vi "Global Parameter.vi"(3 "error in (no error)":errorcluster caption="错误输入（无错误）", 4 "Write":T1, 5 "枚举":enum16{"Inital", "Read", "Write", "Quit"}(ring)) -> (0 "错误输出":errorcluster, 1 "Read":T1)   [LabVIEW 2023]
uses:
  Ctl/Global Parameter.ctl
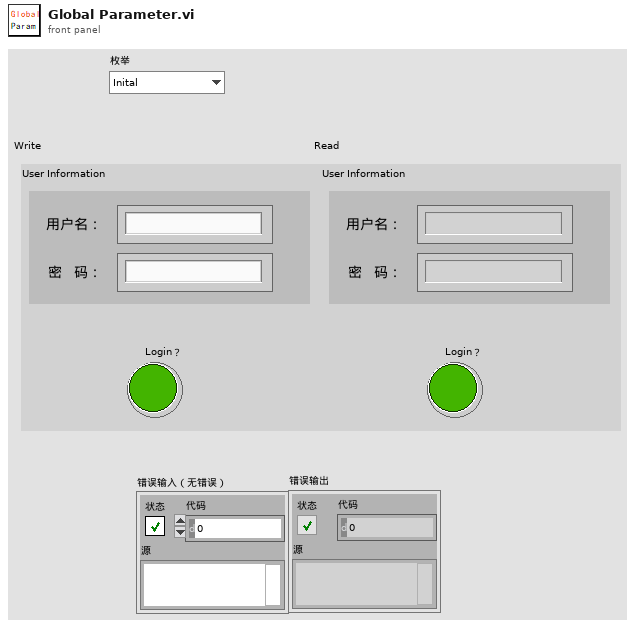
[diagram p1: front panel]
types:
  T1 = typedef "Global Parameter.ctl" = cluster{"User Information":cluster{"用户名：":string, "密   码：":string}, "Login？":bool}
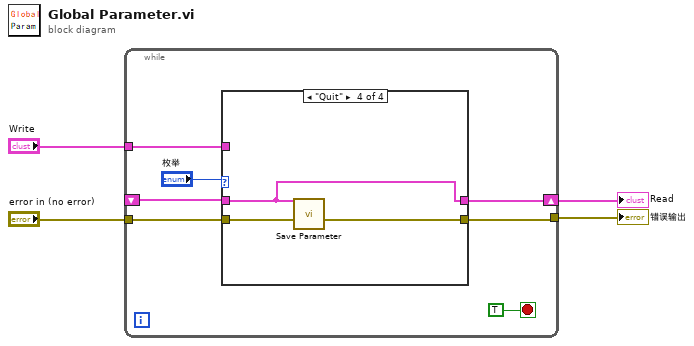
[diagram p0: block diagram]
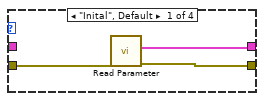
[diagram p2: hidden frame]
diagram:
  n1 = while {
    shift-right: [w8] -> w4
    shift-left: _ -> [w10]
    tunnel: "Write" -> [w9]
    tunnel: "error in (no error)" -> [w7]
    tunnel: [w6] -> w1
    stop <- TRUE stop-if-true
    n2 = case shown="\"Quit\"" "枚举" {
      tunnel: w10 -> [_ w16 _ w19]
      tunnel: w9 -> [_ _ w18 _]
      tunnel: [w14 w16 w18 w19] -> w8
      tunnel: w7 -> [w13 w15 w17 w21]
      tunnel: [w12 w15 w17 w20] -> w6
      frame "Inital", Default {
        n3 = call "Read Parameter.vi"("error in (no error)"=w13) -> ("错误输出"=w12:errorcluster, "Param Out"=w14:T1)  [unwired: 9 in]
      }
      frame "Read" {
      }
      frame "Write" {
      }
      frame "Quit" {
        n4 = call "Save Parameter.vi"("error in (no error)"=w21, "Parameter In"=w19) -> ("error out"=w20:errorcluster)  [unwired: 9 in]
      }
    }
  }
  "Read" <- w4
  "错误输出" <- w1
